vi "Analyze.vi"(8 "error in (no error)":errorcluster, 10 "Threshold (rms)":dbl, 11 "N-Channel Data (2D DBL)":dbl[][](array[numeric])) -> (0 "error out":errorcluster, 1 "Message":string, 2 "Threshold Exceeded?":bool, 3 "N-Channel RMS Results":dbl[](array[numeric]))   [LabVIEW 2020]
uses:
  <vilib>/Analysis/5stat.llb/RMS (DBL).vi
  <vilib>/Analysis/NI_AALPro.lvlib
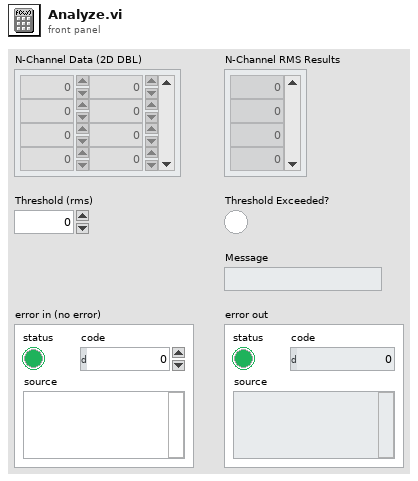
[diagram p1: front panel]
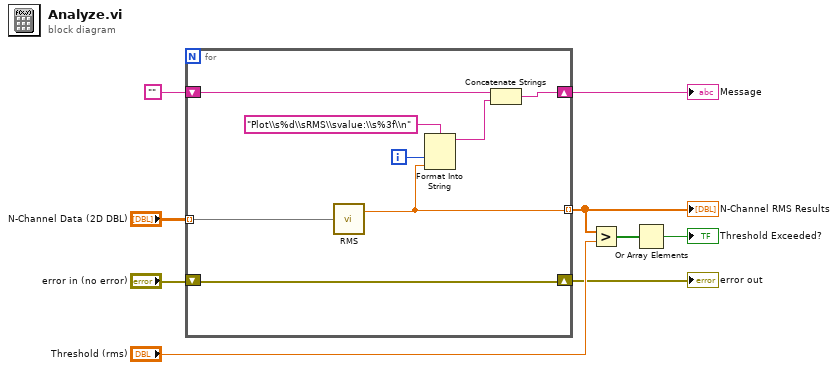
[diagram p0: block diagram]
diagram:
  n1 = for {
    tunnel: [w16] -> w6 mode=indexing
    tunnel: "N-Channel Data (2D DBL)" -> [w15] mode=indexing
    shift-right: [w10] -> w5
    shift-left: "" -> [w11]
    shift-right: [w14] -> w3
    shift-left: "error in (no error)" -> [w14]
    i -> [w17]
    n2 = call-poly <vilib>:"RMS.vi"("X"=w15) -> ("rms value"=w16:dbl)  [unwired: 1 out]
    n3 = Format Into String(format string="Plot\\s%d\\sRMS\\svalue:\\s%3f\\n", w17, w16) -> (resulting string=w12:string)  [unwired: 2 in, 1 out]
    n4 = Concatenate Strings(w11, w12) -> (w10:string)
  }
  "N-Channel RMS Results" <- w6
  "error out" <- w3
  "Message" <- w5
  n5 = Greater?(x=w6, y="Threshold (rms)") -> (0:w8:bool[])
  n6 = Or Array Elements(Boolean array=w8) -> (logical OR=→"Threshold Exceeded?":bool)
